vi "format set num format index.vi"(8 "error in (no error)":errorcluster, 10 "index":u8, 11 "format":u32) -> (0 "error out":errorcluster)   [LabVIEW 8.6]
doc: "void format_set_num_format_index(lxw_format format, uint8_t index);"
uses:
  pending_lvxlsxwriter/xlsxwriter.dll
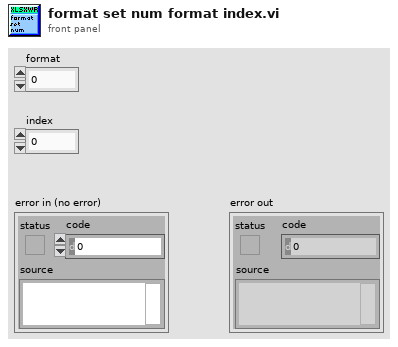
[diagram p1: front panel]
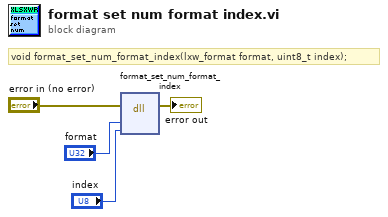
[diagram p0: block diagram]
diagram:
  # "void format_set_num_format_index(lxw_format format, uint8_t index);"
  n1 = dll-call lib="C:/Users/WDAGUtilityAccount/Desktop/pending_lvxlsxwriter/xlsxwriter.*" fn="format_set_num_format_index"(error in="error in (no error)", "format"="format", "index"="index") -> (error out=→"error out":errorcluster)  [unwired: 5 in, 1 out]
